vi "Assignment_02.vi"() -> ()   [LabVIEW 2020]
uses:
  <vilib>/Analysis/3filter.llb/Filter Passband Type.ctl
  <vilib>/Analysis/2dsp.llb/Real FFT.vi
  <vilib>/Analysis/3filter.llb/Butterworth Filter (DBL).vi
  <vilib>/Analysis/3filter.llb/Elliptic Filter (DBL).vi
  <vilib>/Analysis/3filter.llb/Chebyshev Filter (DBL).vi
  <vilib>/Analysis/3filter.llb/Inverse Chebyshev Filter (DBL).vi
  <vilib>/Analysis/3filter.llb/Bessel Filter (DBL).vi
  <vilib>/Analysis/NI_AALBase.lvlib
  <vilib>/Analysis/NI_AALPro.lvlib
panel:
  out "Waveform Graph":cluster{i32, dbl, i32[]}(graph)
  in  "END":bool
  in  "Sampling Rate":dbl
  in  "Attenuation":dbl
  in  "Ripple":dbl
  in  "Order":dbl
  in  "Lower":dbl
  in  "Higher":dbl
  in  "Filter Design":T1(ring)
  in  "Filter Type":T2
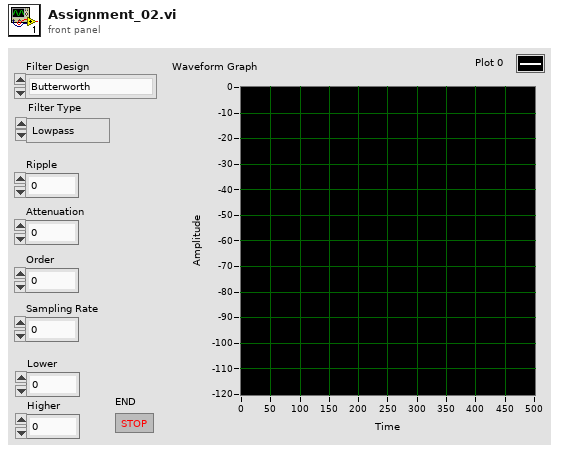
[diagram p1: front panel]
types:
  T1 = enum16{"Butterworth", "Elliptic", "Chebyshev", "Inv Chebyshev", "Bessel"}
  T2 = typedef "NI_AALBase.lvlib/Filter Passband Type.ctl" = enum32{"Lowpass", "Highpass", "Bandpass", "Bandstop"}
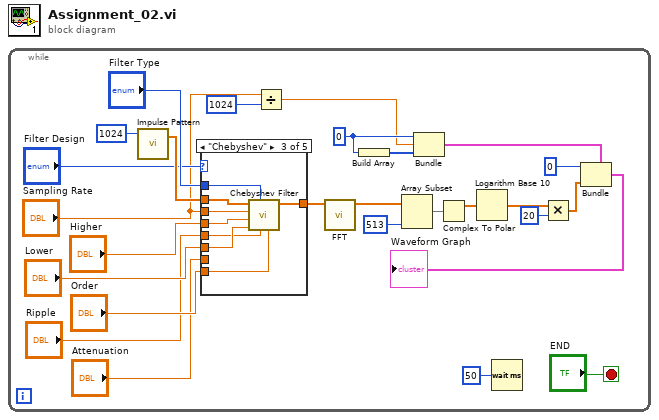
[diagram p0: block diagram]
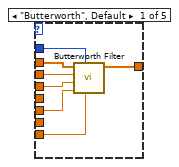
[diagram p2: hidden frame]
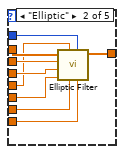
[diagram p3: hidden frame]
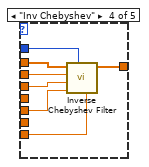
[diagram p4: hidden frame]
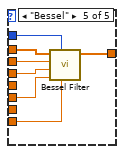
[diagram p5: hidden frame]
diagram:
  n1 = while {
    stop <- "END" stop-if-true
    w4 = 0
    n2 = call <vilib>:"Impulse Pattern.vi"("samples"=1024) -> ("Impulse Pattern"=w23:dbl[])  [unwired: 2 in, 1 out]
    n3 = case shown="\"Chebyshev\"" "Filter Design" {
      tunnel: "Filter Type" -> [w34 w43 w51 w58 w65]
      tunnel: "Higher" -> [w31 w42 w48 w57 w62]
      tunnel: "Lower" -> [w30 w41 w47 w55 w61]
      tunnel: "Order" -> [w29 w40 w45 w54 w60]
      tunnel: "Sampling Rate" -> [w32 w39 w49 w56 w63]
      tunnel: w23 -> [w33 w38 w50 w53 w64]
      tunnel: [w28 w37 w44 w52 w59] -> w21
      tunnel: "Attenuation" -> [_ w36 _ _ _]
      tunnel: "Ripple" -> [_ w35 w46 _ _]
      frame "Butterworth", Default {
        n4 = call-poly <vilib>:"Butterworth Filter.vi"("order"=w29, "filter type"=w34, "low cutoff freq: fl"=w30, "high cutoff freq: fh"=w31, "sampling freq: fs"=w32, "X"=w33) -> ("Filtered X"=w28:dbl[])  [unwired: 2 in, 1 out]
      }
      frame "Elliptic" {
        n5 = call-poly <vilib>:"Elliptic Filter.vi"("order"=w40, "filter type"=w43, "stopband attenuation (dB)"=w36, "passband ripple (dB)"=w35, "low cutoff freq: fl"=w41, "high cutoff freq: fh"=w42, "sampling freq: fs"=w39, "X"=w38) -> ("Filtered X"=w37:dbl[])  [unwired: 2 in, 1 out]
      }
      frame "Chebyshev" {
        n6 = call-poly <vilib>:"Chebyshev Filter.vi"("order"=w45, "ripple(dB)"=w46, "filter type"=w51, "low cutoff freq: fl"=w47, "high cutoff freq: fh"=w48, "sampling freq: fs"=w49, "X"=w50) -> ("Filtered X"=w44:dbl[])  [unwired: 3 in, 1 out]
      }
      frame "Inv Chebyshev" {
        n7 = call-poly <vilib>:"Inverse Chebyshev Filter.vi"("order"=w54, "filter type"=w58, "low cutoff freq: fl"=w55, "high cutoff freq: fh"=w57, "sampling freq: fs"=w56, "X"=w53) -> ("Filtered X"=w52:dbl[])  [unwired: 4 in, 1 out]
      }
      frame "Bessel" {
        n8 = call-poly <vilib>:"Bessel Filter.vi"("order"=w60, "filter type"=w65, "low cutoff freq: fl"=w61, "high cutoff freq: fh"=w62, "sampling freq: fs"=w63, "X"=w64) -> ("Filtered X"=w59:dbl[])  [unwired: 2 in, 1 out]
      }
    }
    n9 = Divide(x="Sampling Rate", y=1024) -> (x/y=w2:dbl)
    n10 = call-poly <vilib>:"FFT.vi"("X"=w21) -> ("FFT {X}"=w17:cdb[])  [unwired: 9 in, 1 out]
    n11 = Build Array(w4) -> (w3:i32[])
    n12 = Array Subset(array=w17, length=513) -> (w15:cdb[])  [unwired: 1 in]
    n13 = Bundle(w4, w2, w3) -> (w1:cluster{i32, dbl, i32[]})  [unwired: 1 in]
    n14 = Complex To Polar(r * e^(i*theta)=w15) -> (r=w12:dbl[])  [unwired: 1 out]
    n15 = Logarithm Base 10(1:w12) -> (0:w13:dbl[])
    n16 = Wait (ms)(milliseconds to wait=50) -> ()  [unwired: 1 out]
    n17 = Multiply(x=w13, y=20) -> (x*y=w11:dbl[])
    n18 = Bundle(cluster=w1, 0, w11) -> (→"Waveform Graph":cluster{i32, dbl, i32[]})  [unwired: 1 in]
  }
